vi "Get Slide Size.vi"() -> (8 "Slide Size Out mm)":dbl format="%#_4g")   [LabVIEW 2016]
uses:
  <vilib>/Utility/miscctls.llb/LVPointTypeDef.ctl
panel:
  in  "Okay":bool
  in  "Slide Size (mm)":dbl format="%#_4g"
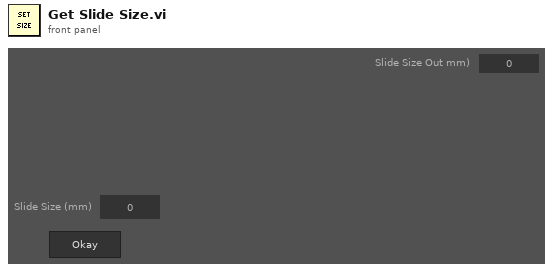
[diagram p1: front panel]
types:
  T1 = enum16{"Always On", "Always Off", "Off While Running"}
  T2 = typedef "LVPointTypeDef.ctl" = cluster{"Horizontal":i16, "Vertical":i16}
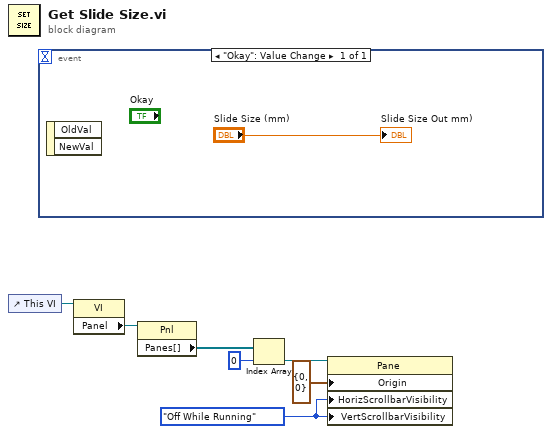
[diagram p0: block diagram]
diagram:
  w1 = T1."Off While Running" ("Vertical Scrollbar Visibility")
  n1 = control-ref of="This VI"() -> (w7:refnum<vi>)
  n2 = event shown="[0] \"Okay\": Value Change" {
    selector: _ -> [_]
    dyn-events: _ -> [_]
    timeout: _ -> [_]
    event "Okay": Value Change {
      n3 = event-data() -> ()  [unwired: 1 in, 2 out]
      "Slide Size Out mm)" <- "Slide Size (mm)"
    }
  }
  n4 = property class="VI"(reference=w7) -> ("Panel"=w6:refnum<vi>)  [unwired: 1 in, 2 out]
  n5 = property class="Pnl"(reference=w6) -> ("Panes[]"=w3:refnum<vi>[])  [unwired: 1 in, 2 out]
  n6 = Index Array(array=w3, index=0) -> (element=w4:refnum<vi>)
  n7 = property class="Pane"(reference=w4, "Origin"=T2 {"Horizontal"=0, "Vertical"=0}, "HorizScrollbarVisibility"=w1, "VertScrollbarVisibility"=w1) -> ()  [unwired: 1 in, 2 out]
